vi "CreatePublicEvents.vi"(8 "error in (no error)":errorcluster, 11 "DAQmx":refnum<class "DAQmx.lvclass">) -> (0 "error out":errorcluster, 3 "DAQmx out":refnum<class "DAQmx.lvclass">)   [LabVIEW 2019, in "DAQmx.lvclass"]
uses:
  DAQmx.lvclass
  typedefs/DAQmx.Status--enum.ctl
  typedefs/DeviceInfo--Cluster.ctl
  typedefs/DAQ.Config.AO--Cluster--Array.ctl
  typedefs/DAQ.Config.AO--Cluster.ctl
  typedefs/DAQ.Config.AO.Range--enum.ctl
  typedefs/DAQ.Config.Device Type--enum.ctl
  typedefs/DAQ.Config.AI--Cluster--Array.ctl
  typedefs/DAQ.Config.AI--Cluster.ctl
  typedefs/DAQ.Config.AI.Coupling--enum.ctl
  typedefs/DAQ.Config.AI.Range--enum.ctl
  typedefs/DAQ.Config.Timing--Cluster.ctl
  typedefs/DAQ.Config.Timing.Sampling--Cluster.ctl
  typedefs/DAQ.Config.Timing.Fs Mode--enum.ctl
  typedefs/PrivateEvent--Waveforms--cluster.ctl
  DAQmx.lvclass/DAQmx.ctl
  <vilib>/JKI/JKI SMO/SMO/SMO.lvclass
panel:
  # "For instructions on how to use the JKI State Machine Objects, examples and video tutorials, visit:\nhttp://jki.net/state-machine-objects/\n\nJKI State Machine Objects™\nhttp://jki.net/state-machine-objects/\nCopyright (C) 2005-2015, JKI <info@jki.net>\nALL RIGHTS RESERVED"
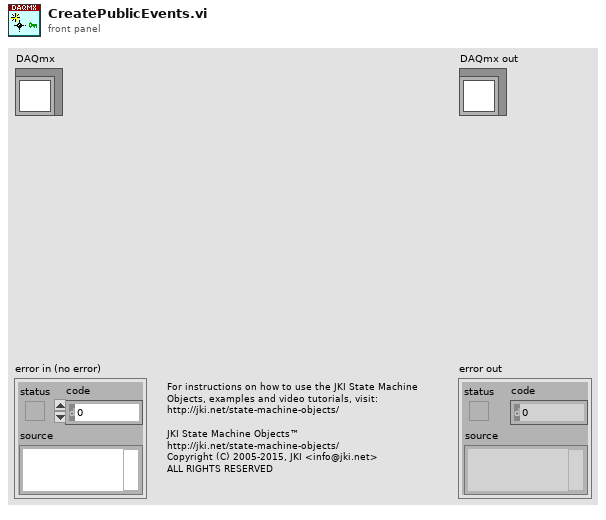
[diagram p1: front panel]
types:
  T1 = cluster{"Active Device":string, "SelfCal.LastDate/Time":string, "SelfCal.LastTemp":dbl, "DevTemp":dbl, "calibration due?":bool}[]
  T2 = typedef "DAQmx.lvclass/PrivateEvent--Waveforms--cluster.ctl" = cluster{"AO":waveform(dbl)[], "AI":waveform(dbl)[], "REF_X":waveform(dbl)[], "REF_Y":waveform(dbl)[]}
  T3 = typedef "DAQmx.lvclass/DAQ.Config.Timing--Cluster.ctl" = cluster{"Sampling":T4, "sample mode":i32, "FsMode":T5, "Fs Multiplier":dbl, "Refresh Rate (Hz)":dbl, "Decimation.PreDSP":i32, "Decimation.PostDSP":i32, "Fs.Output":dbl}
  T4 = typedef "DAQmx.lvclass/DAQ.Config.Timing.Sampling--Cluster.ctl" = cluster{"Fs":dbl, "#s":i32}
  T5 = typedef "DAQmx.lvclass/DAQ.Config.Timing.Fs Mode--enum.ctl" = enum16{"Manual", "Auto Fs", "Max Fs"}
  T6 = typedef "DAQmx.lvclass/DAQ.Config.AI--Cluster--Array.ctl" = T7[]
  T7 = typedef "DAQmx.lvclass/DAQ.Config.AI--Cluster.ctl" = cluster{"Channels":tag, "Coupling":T8, "Range":T9, "input terminal configuration":i32, "Type":T10}
  T8 = typedef "DAQmx.lvclass/DAQ.Config.AI.Coupling--enum.ctl" = u16
  T9 = typedef "DAQmx.lvclass/DAQ.Config.AI.Range--enum.ctl" = enum16{"±0.316", "±1.00", "±3.16", "±10.0", "±31.6", "±42.4", ""}
  T10 = typedef "DAQmx.lvclass/DAQ.Config.Device Type--enum.ctl" = enum16{"None", "USB-4431", "PXI-446x"}
  T11 = typedef "DAQmx.lvclass/DAQ.Config.AO--Cluster--Array.ctl" = T12[]
  T12 = typedef "DAQmx.lvclass/DAQ.Config.AO--Cluster.ctl" = cluster{"Channels":tag, "Range":T13, "output terminal configuration":i32, "Type":T10}
  T13 = typedef "DAQmx.lvclass/DAQ.Config.AO.Range--enum.ctl" = enum16{"±0.1", "±1.0", "±3.5", "±10.0", ""}
  T14 = typedef "DAQmx.lvclass/DeviceInfo--Cluster.ctl" = cluster{"DeviceName":string, "DevIsSimulated":bool, "DeviceSerialNumber":string, "ProductType":string, "ProductCategory":i32, "ProductNumber":u32, "ChassisNumber":u32, "SlotNumber":u32, "ChassisName":string, "ChassisSerialNumber":string, "DevTemp":dbl, "SelfCal.LastDate/Time":string, "SelfCal.LastTemp":dbl, "calibration due?":bool}
  T15 = typedef "DAQmx.lvclass/DAQmx.Status--enum.ctl" = enum16{"idle", "calibrating", "configuring", "creating", "created", "starting", "started", "stopping", "stopped", "clearing", "error"}
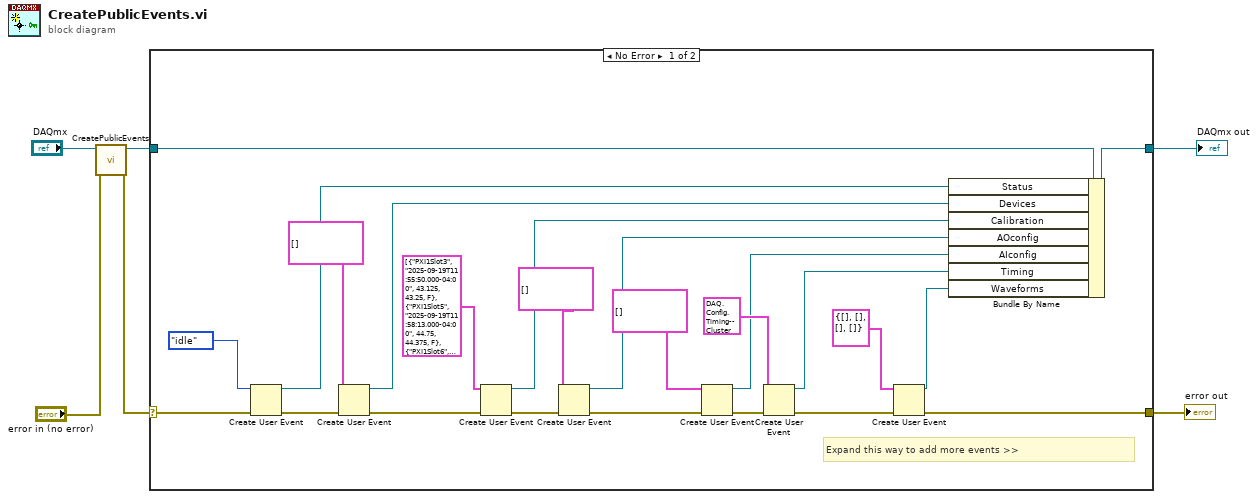
[diagram p0: block diagram]
diagram:
  n1 = call-parent "CreatePublicEvents.vi"("error in (no error)"="error in (no error)", "SMO"="DAQmx") -> ("error out"=w1:errorcluster, "SMO out"=w5:refnum<class "DAQmx.lvclass">)  [unwired: 8 in]
  n2 = case shown="No Error" w1 {
    selector: w1 -> [w28 w32]
    tunnel: [w11 w32] -> w3
    tunnel: [w30 w31] -> w4
    tunnel: w5 -> [w26 w31]
    frame No Error {
      # "Expand this way to add more events >>"
      n3 = Create User Event(user event datatype=DAQmx.Status--enum."idle" ("Status"), error in=w28) -> (user event=w27:refnum<user-event>, error out=w18:errorcluster)
      n4 = Create User Event(user event datatype=T14[] [] ("event data"), error in=w18) -> (user event=w19:refnum<user-event>, error out=w13:errorcluster)
      n5 = Create User Event(user event datatype=T1 [{"Active Device"="PXI1Slot3", "SelfCal.LastDate/Time"="2025-09-19T11:55:50.000-04:00", "SelfCal.LastTemp"=43.125, "DevTemp"=43.25, "calibration due?"=FALSE}, {"Active Device"="PXI1Slot5", "SelfCal.LastDate/Time"="2025-09-19T11:58:13.000-04:00", "SelfCal.LastTemp"=44.75, "DevTemp"=44.375, "calibration due?"=FALSE}, {"Active Device"="PXI1Slot6", "SelfCal.LastDate/Time"="2025-09-19T12:00:36.000-04:00", "SelfCal.LastTemp"=45.625, "DevTemp"=45.0, "calibration due?"=FALSE}, {"Active Device"="PXI1Slot7", "SelfCal.LastDate/Time"="2025-09-19T12:02:59.000-04:00", "SelfCal.LastTemp"=45.125, "DevTemp"=45.25, "calibration due?"=FALSE}, {"Active Device"="PXI1Slot8", "SelfCal.LastDate/Time"="2025-09-19T12:05:22.000-04:00", "SelfCal.LastTemp"=49.125, "DevTemp"=49.375, "calibration due?"=FALSE}] ("Calibration out"), error in=w13) -> (user event=w7:refnum<user-event>, error out=w12:errorcluster)
      n6 = Create User Event(user event datatype=T11 [] ("event data"), error in=w12) -> (user event=w20:refnum<user-event>, error out=w17:errorcluster)
      n7 = Create User Event(user event datatype=T6 [] ("event data"), error in=w17) -> (user event=w14:refnum<user-event>, error out=w16:errorcluster)
      n8 = Create User Event(user event datatype=T3 {"Sampling"={"Fs"=1000.0, "#s"=128}, "sample mode"=10123, "FsMode"=enum."Manual", "Fs Multiplier"=1.0, "Refresh Rate (Hz)"=10.0, "Decimation.PreDSP"=1, "Decimation.PostDSP"=1, "Fs.Output"=204789.0} ("event data"), error in=w16) -> (user event=w21:refnum<user-event>, error out=w15:errorcluster)
      n9 = Create User Event(user event datatype=T2 {"AO"=[], "AI"=[], "REF_X"=[], "REF_Y"=[]} ("Waveforms"), error in=w15) -> (user event=w9:refnum<user-event>, error out=w11:errorcluster)
      n10 = Bundle By Name(cluster=w26, "Status"=w27, "Devices"=w19, "Calibration"=w7, "AOconfig"=w20, "AIconfig"=w14, "Timing"=w21, "Waveforms"=w9) -> (w30:refnum<class "DAQmx.lvclass">)
    }
    frame Error {
    }
  }
  "error out" <- w3
  "DAQmx out" <- w4
